vi "fpga_InputOverflowOR.vi"(1 "Input Lines":T1, 2 "overflow":bool) -> (0 "Output Lines":T1)   [LabVIEW 2011]
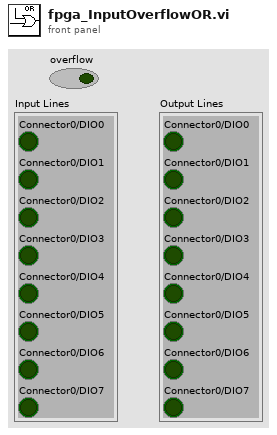
[diagram p1: front panel]
types:
  T1 = cluster{"Connector0/DIO0":bool, "Connector0/DIO1":bool, "Connector0/DIO2":bool, "Connector0/DIO3":bool, "Connector0/DIO4":bool, "Connector0/DIO5":bool, "Connector0/DIO6":bool, "Connector0/DIO7":bool}
  T2 = cluster{bool, bool, bool, bool, bool, bool, bool, bool}
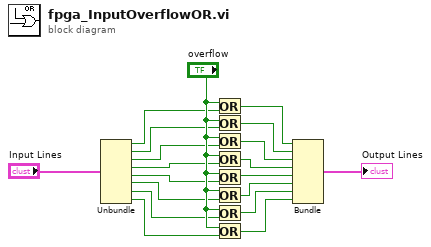
[diagram p0: block diagram]
diagram:
  n1 = Unbundle("Input Lines") -> ("Connector0/DIO0"=w9:bool, "Connector0/DIO1"=w8:bool, "Connector0/DIO2"=w7:bool, "Connector0/DIO3"=w6:bool, "Connector0/DIO4"=w5:bool, "Connector0/DIO5"=w2:bool, "Connector0/DIO6"=w3:bool, "Connector0/DIO7"=w4:bool)
  n2 = Or(x="overflow", y=w9) -> (x .or. y?=w17:bool)
  n3 = Or(x="overflow", y=w8) -> (x .or. y?=w16:bool)
  n4 = Or(x="overflow", y=w7) -> (x .or. y?=w15:bool)
  n5 = Or(x="overflow", y=w6) -> (x .or. y?=w14:bool)
  n6 = Or(x="overflow", y=w5) -> (x .or. y?=w13:bool)
  n7 = Or(x="overflow", y=w2) -> (x .or. y?=w12:bool)
  n8 = Or(x="overflow", y=w3) -> (x .or. y?=w11:bool)
  n9 = Or(x="overflow", y=w4) -> (x .or. y?=w10:bool)
  n10 = Bundle(w17, w16, w15, w14, w13, w12, w11, w10) -> (→"Output Lines":T2)  [unwired: 1 in]
